vi "Build Command.vi"(5 "Target":u8, 7 "CMD ID":u8, 8 "error in (no error)":errorcluster, 9 "Data 3":u16 format="%04x", 10 "Data 2":u16 format="%04x", 11 "Data 1":u16 format="%04x") -> (0 "error out":errorcluster, 2 "Command":u64)   [LabVIEW 2020, in "BCI-1553 API.lvlib" / "FPGA Interface.lvlib" / "FPGA Interface.lvclass"]
doc: "Builds a standard command that can be sent to a component in the 1553 Session."
uses:
  FPGA Interface.lvclass
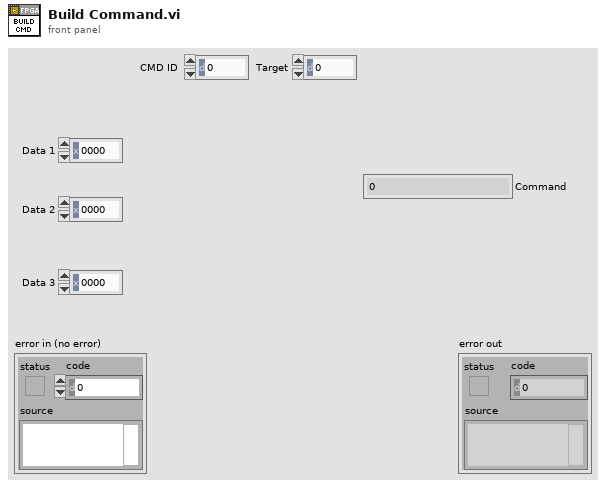
[diagram p1: front panel]
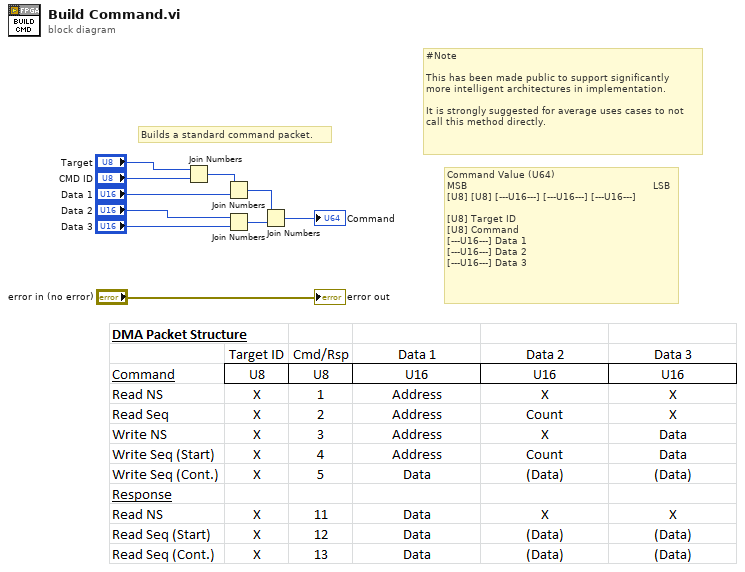
[diagram p0: block diagram]
diagram:
  # "Command Value (U64)\nMSB                                                              LSB\n[U8] [U8] [---U16---] [---U16---] [---U16---]\n\n[U8] Target ID\n[U8] Command\n[---U16---] Data 1\n[---U16---] Data 2\n[---U16---] Data 3"
  # "#Note\n\nThis has been made public to support significantly\nmore intelligent architectures in implementation.\n\nIt is strongly suggested for average uses cases to not\ncall this method directly."
  # "Builds a standard command packet."
  n1 = Join Numbers(hi="Target", lo="CMD ID") -> ((hi.lo)=w7:u16)
  n2 = Join Numbers(hi=w7, lo="Data 1") -> ((hi.lo)=w6:u32)
  n3 = Join Numbers(hi="Data 2", lo="Data 3") -> ((hi.lo)=w3:u32)
  n4 = Join Numbers(hi=w6, lo=w3) -> ((hi.lo)=→"Command":u64)
  "error out" <- "error in (no error)"
